vi "2.6.-Lectura de Video.vi"() -> ()   [LabVIEW 2020]
uses:
  <vilib>/userDefined/High Color/IMAQdx.ctl
  <vilib>/vision/driver/NI_Vision_Acquisition_Software.lvlib
panel:
  in  "IMAQdx Session":T1
  out "Image":T2(plugin-control)
  in  "stop":bool
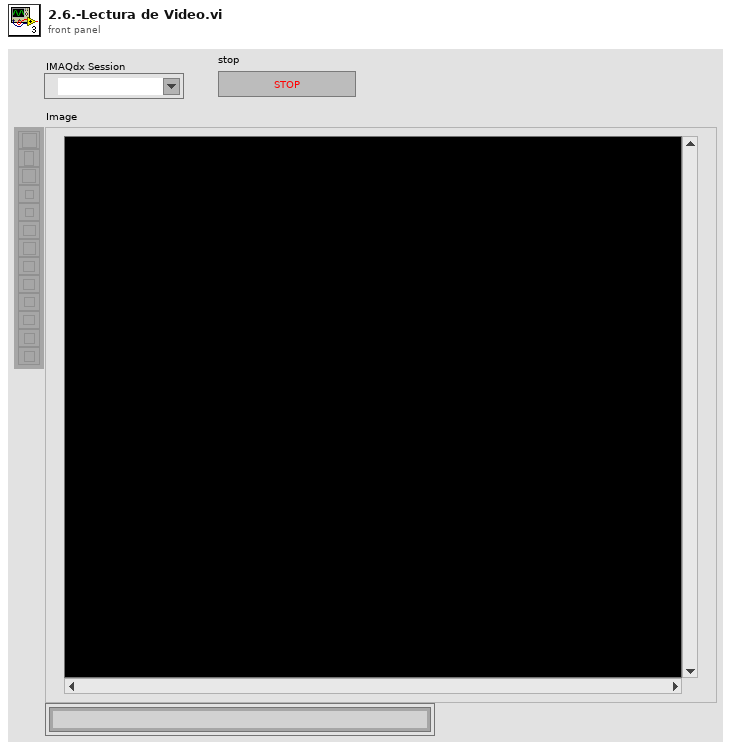
[diagram p1: front panel]
types:
  T1 = typedef "IMAQdx.ctl" = refnum<k21>
  T2 = typedef "IMAQ Image.ctl" = refnum<image>
  T3 = typedef "Image Type" = u32
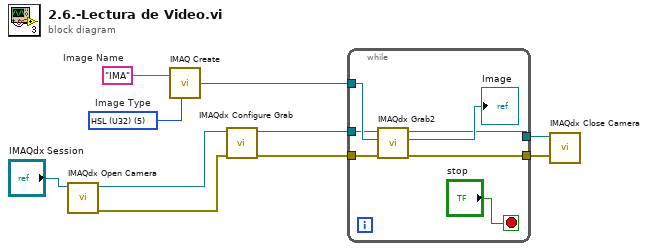
[diagram p0: block diagram]
diagram:
  w1 = "IMA"  # Image Name
  w2 = T3 5 items=["Grayscale (U8)", "Grayscale (I16)", "Grayscale (SGL)", "Complex (CSG)", "RGB (U32)", "HSL (U32)", "RGB (U64)", "Grayscale (U16)"]  # Image Type
  n1 = call <vilib>:"IMAQdx Open Camera.vi"("Session In"="IMAQdx Session") -> ("error out"=w8:errorcluster, "Session Out"=w9:T1)  [unwired: 9 in]
  n2 = call "IMAQ Create"("Image Name"=w1, "Image Type"=w2) -> ("New Image"=w7:T2)  [unwired: 3 in, 1 out]
  n3 = call <vilib>:"IMAQdx Configure Grab.vi"("error in"=w8, "Session In"=w9) -> ("error out"=w5:errorcluster, "Session Out"=w6:T1)  [unwired: 8 in]
  n4 = while {
    tunnel: w7 -> [w15]
    tunnel: w6 -> [w14]
    tunnel: w5 -> [w16]
    tunnel: [w11] -> w4
    tunnel: [w13] -> w3
    stop <- "stop" stop-if-true
    n5 = call <vilib>:"IMAQdx Grab2.vi"("error in"=w16, "Image In"=w15, "Session In"=w14) -> ("error out"=w13:errorcluster, "Image Out"=→"Image":T2, "Session Out"=w11:T1)  [unwired: 5 in, 1 out]
  }
  n6 = call <vilib>:"IMAQdx Close Camera.vi"("error in"=w3, "Session In"=w4) -> ()  [unwired: 9 in, 1 out]
